vi "close.vi"(8 "error in (no error)":errorcluster, 11 "Template Action Runtime in":refnum<class "Template Action Runtime.lvclass">) -> (0 "error out":errorcluster, 3 "Template Action Runtime out":refnum<class "Template Action Runtime.lvclass">)   [LabVIEW 2014, in "Template Action Runtime.lvclass"]
uses:
  Template Action Runtime.lvclass
  <vilib>/NI/TBM Modules/Sequencer/sequencer parent classes/action parent/action.lvclass
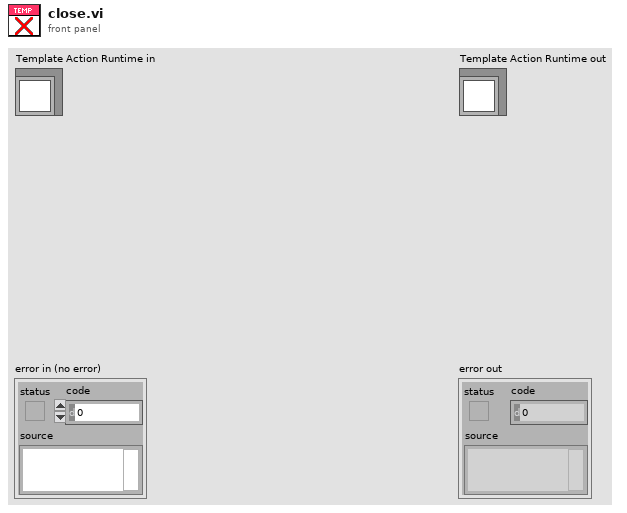
[diagram p1: front panel]
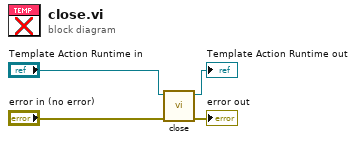
[diagram p0: block diagram]
diagram:
  n1 = call-parent "close.vi"("error in (no error)"="error in (no error)", "action in"="Template Action Runtime in") -> ("error out"=→"error out":errorcluster, "action out"=→"Template Action Runtime out":refnum<class "Template Action Runtime.lvclass">)  [unwired: 8 in]
